vi "Delete Int64Array DVR.vi"(8 "error in (no error)":errorcluster, 11 "Int64Array DVR in":refnum<data-value>) -> (0 "error out":errorcluster, 3 "Int64Array out":refnum<class "Int64Array.lvclass">)   [LabVIEW 2012, in "MDSplus.lvlib" / "Int64Array.lvclass"]
uses:
  <vilib>/MDSplus/Classes/Data_Class/Array_Class/Int64Array_Class/Int64Array.lvclass
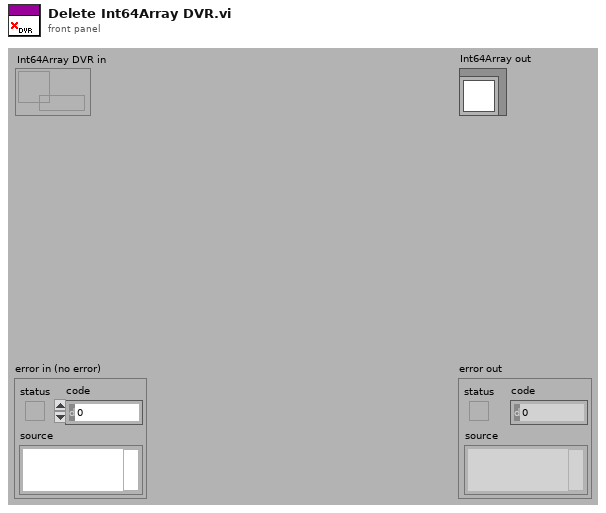
[diagram p1: front panel]
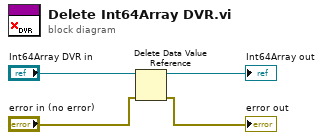
[diagram p0: block diagram]
diagram:
  n1 = Delete Data Value Reference(data value reference="Int64Array DVR in", error in="error in (no error)") -> (data value=→"Int64Array out":refnum<class "Int64Array.lvclass">, error out=→"error out":errorcluster)
